vi "Main.vi"(7 "GenNet Protocol":refnum<class "GenNet Protocol.lvclass">, 9 "Port Number":u16, 10 "Caller MsgQ":refnum<class "DQMH-GenNet Message Queue.lvclass">, 11 "Module Admin":refnum<class "Delacor_lib_QMH_Cloneable Module Admin.lvclass">) -> ()   [LabVIEW 2020, in "GenNet-Server.lvlib"]
doc: "The GenNet-Server module is instantiated from a DQMH Generic Networking Module\nin order to accept messages via TCP/IP. \n\nThe GenNet-Server module accepts messages from any DQMH Generic Networking \nModule running in another application and/or on another PC.\n\n<b>Note:</b> This VI was modified by the <b>Validate DQMH Module</b> tool to upgrade it to the DQMH 5.0 approach to destroying cloneable module event references.\n\n<b>Note:</b> This VI was modified by the <b>Validate DQMH Module</b> tool to have the module name be passed as the Additional Information parameter with an Error Reported broadcast.\n\n<b>Note:</b> This VI was modified by the <b>Validate DQMH Module</b> tool to call the Release Message Queue VI in the top-level Error case.\n\n<b>Note:</b> This VI was modified by the <b>Validate DQMH Module</b> tool to call the Release Message Queue VI in the top-level Error case.\n\n<b>Note:</b> This VI was modified by the <b>Validate DQMH Module</b> tool to add a call to the Error Reported VI at the end of the 'Exit' MHL frame.\n\n____\nHAMPEL SOFTWARE ENGINEERING v3.8.0 (2023-12-18 14:41)"
uses:
  GenNet-Server.lvlib
  <vilib>/Delacor/Delacor QMH/Libraries/Cloneable Module Admin_class/Delacor_lib_QMH_Cloneable Module Admin.lvclass
  C:/Program Files (x86)/National Instruments/LabVIEW 2020/vi.lib/Delacor/Delacor QMH/Libraries/Module Admin_class/Delacor_lib_QMH_Module Admin.lvclass
  DQMH-GenNet Message Queue.lvclass
  GenNet Protocols/GenNet Protocol.lvclass
  SubVIs/TCP_Comm-States.ctl
  UDP Broadcasting/Generic Broadcasts.ctl
  hse-dqmh/Dynamic Requesters/Singleton/Status Updated Argument--cluster.ctl
  hse-dqmh/Dynamic Requesters/Singleton/Error Reported Argument--cluster.ctl
  hse-dqmh/Dynamic Requesters/Singleton/Get Module Execution Status Argument--cluster.ctl
  hse-dqmh/Dynamic Requesters/Singleton/Stop Argument--cluster.ctl
  hse-dqmh/Controls/System Message Argument--cluster.ctl
  hse-dqmh/Controls/System Message Source.ctl
  Module Data--cluster.ctl
  UDP Broadcasting/Network Broadcast Params.ctl
  Stop Argument--cluster.ctl
  <vilib>/Delacor/Delacor QMH/Libraries/Message Queue_class/Delacor_lib_QMH_Message Queue.lvclass/Delacor_lib_QMH_Message Queue.ctl
  UDP Broadcasting/Broadcast Arguments/Error Reported - Arguments.ctl
  UDP Broadcasting/Broadcast Arguments/Module Did Stop - Arguments.ctl
  Forward Generic Broadcasts to Network Argument--cluster.ctl
  <vilib>/Delacor/Delacor QMH/Libraries/Cloneable Module Admin_class/Delacor_lib_QMH_Cloneable Module Admin.lvclass/Delacor_lib_QMH_Cloneable Module Admin.ctl
  <vilib>/Delacor/Delacor QMH/Libraries/Module Admin_class/Delacor_lib_QMH_Module Admin.lvclass/Delacor_lib_QMH_Module Admin.ctl
  <vilib>/Utility/miscctls.llb/LVPointTypeDef.ctl
  <vilib>/Delacor/Delacor QMH/Libraries/Cloneable Module Admin_class/Delacor_lib_QMH_Get Module ID.vi
  <vilib>/Delacor/Delacor QMH/Libraries/Message Queue_class/Delacor_lib_QMH_Enqueue Message (Single).vi
  <vilib>/Delacor/Delacor QMH/Libraries/Module Admin_class/Delacor_lib_QMH_Get External Launch.vi
  <vilib>/Utility/tcp.llb/UDP Multicast Write-Only Open.vi
  <vilib>/Utility/error.llb/Error Cluster From Error Code.vi
  <vilib>/ErrorRing/Error Ring.xnode
  <vilib>/Delacor/Delacor QMH/Libraries/Message Queue_class/Delacor_lib_QMH_Message Queue.lvclass
  hse-dqmh/hse-dqmh.lvlib
  hse-gennet.lvlib
  hse-dqmh/hse-dqmh-dynamicrequesters.lvlib
panel:
  out "listener ID":refnum<k5>
  out "error out":errorcluster
  # "The GenNet Protocol allows for injecting the actual protocol (or, rather, the format\nor encoding used for the TCP messages). This also defines how to handle incoming\nmessages (eg. write them directly to the Caller MsgQ or broadcast them)"
  # "The GenNet-Server module is instantiated from a DQMH Generic Networking Module\n(the caller) in order to accept messages via TCP/IP. \n\nThe GenNet-Server module accepts messages from any DQMH Generic Networking \nModule running in another application and/or on another PC."
  # "Caveat:\nThe Caller's message queue, which should be private to the caller only, is avail-\nable to the GenNet-Server module so that it can write messages directly. As the GenNet-Server\nmodule cannot be accessed from other code, and as messages that arrive via\nnetwork are to be considered local, this excemption to the rule is tolerable."
  # "Please get in touch with us at office@hampel-soft.com or visit our website www.hampel-soft.com"
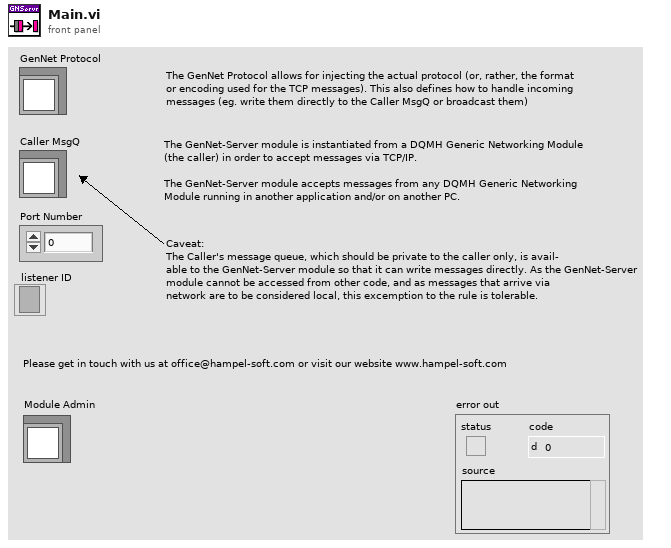
[diagram p1: front panel]
types:
  T1 = typedef "hse-gennet.lvlib/Generic Broadcasts.ctl" = cluster{"Status Updated":refnum<user-event>, "Error Reported":refnum<user-event>, "Update Module Execution Status":refnum<user-event>, "Module Did Stop":refnum<user-event>, "System Message":refnum<user-event>}
  T2 = typedef "GenNet-Server.lvlib/TCP_Comm-States.ctl" = enum16{"Idle", "Open port", "Wait for connection...", "Close port"}
  T3 = typedef "GenNet-Server.lvlib/Request Events--cluster.ctl" = cluster{"Stop Module":refnum<user-event>, "Show Panel":refnum<user-event>, "Hide Panel":refnum<user-event>, "Show Diagram":refnum<user-event>, "Get Module Execution Status":refnum<user-event>, "Forward Generic Broadcasts to Network":refnum<user-event>}
  T4 = typedef "GenNet-Server.lvlib/Module Data--cluster.ctl" = cluster{"Status":string, "UDP Conn. ID":refnum<k16>, "Network Broadcast Params":T5}
  T5 = typedef "hse-gennet.lvlib/Network Broadcast Params.ctl" = cluster{"Server (Sender) Port":u16, "Client (Receiver) Port":u16, "Multicast Address":string, "Local IP Address":string, "Max Rx Byte Size":i32}
  T6 = enum32{"invalid lock state", "Not Locked", "Locked (No Password)", "Password-protected"}
  T7 = typedef "GenNet-Server.lvlib/Stop Argument--cluster.ctl" = cluster{"Origin":string, "Module ID":i32, "Exit via Stop Module Req?":bool, "Wait for Module to stop?":bool}
  T8 = typedef "hse-gennet.lvlib/Error Reported - Arguments.ctl" = cluster{"Error":errorcluster, "Additional Information":string, "Module Name":string}
  T9 = typedef "hse-gennet.lvlib/Module Did Stop - Arguments.ctl" = cluster{"Origin":string, "Exit via Stop Module Req?":bool, "Wait for Module to stop?":bool}
  T10 = typedef "hse-dqmh.lvlib/System Message Source.ctl" = enum16{"module", "application", "network"}
  T11 = typedef "hse-dqmh.lvlib/System Message Argument--cluster.ctl" = cluster{"Identifier":string, "Payload":variant, "Sys. Msg. Source":T10, "Sys. Msg. Origin":string}
  T12 = typedef "GenNet-Server.lvlib/Forward Generic Broadcasts to Network Argument--cluster.ctl" = cluster{"Module ID":i32, "Generic Broadcast Events":T1, "Network Broadcast Params":T5}
  T13 = typedef "LVPointTypeDef.ctl" = cluster{"Horizontal":i16, "Vertical":i16}
  T14 = enum32{"Invalid", "Standard", "Closed", "Hidden", "Minimized", "Maximized"}
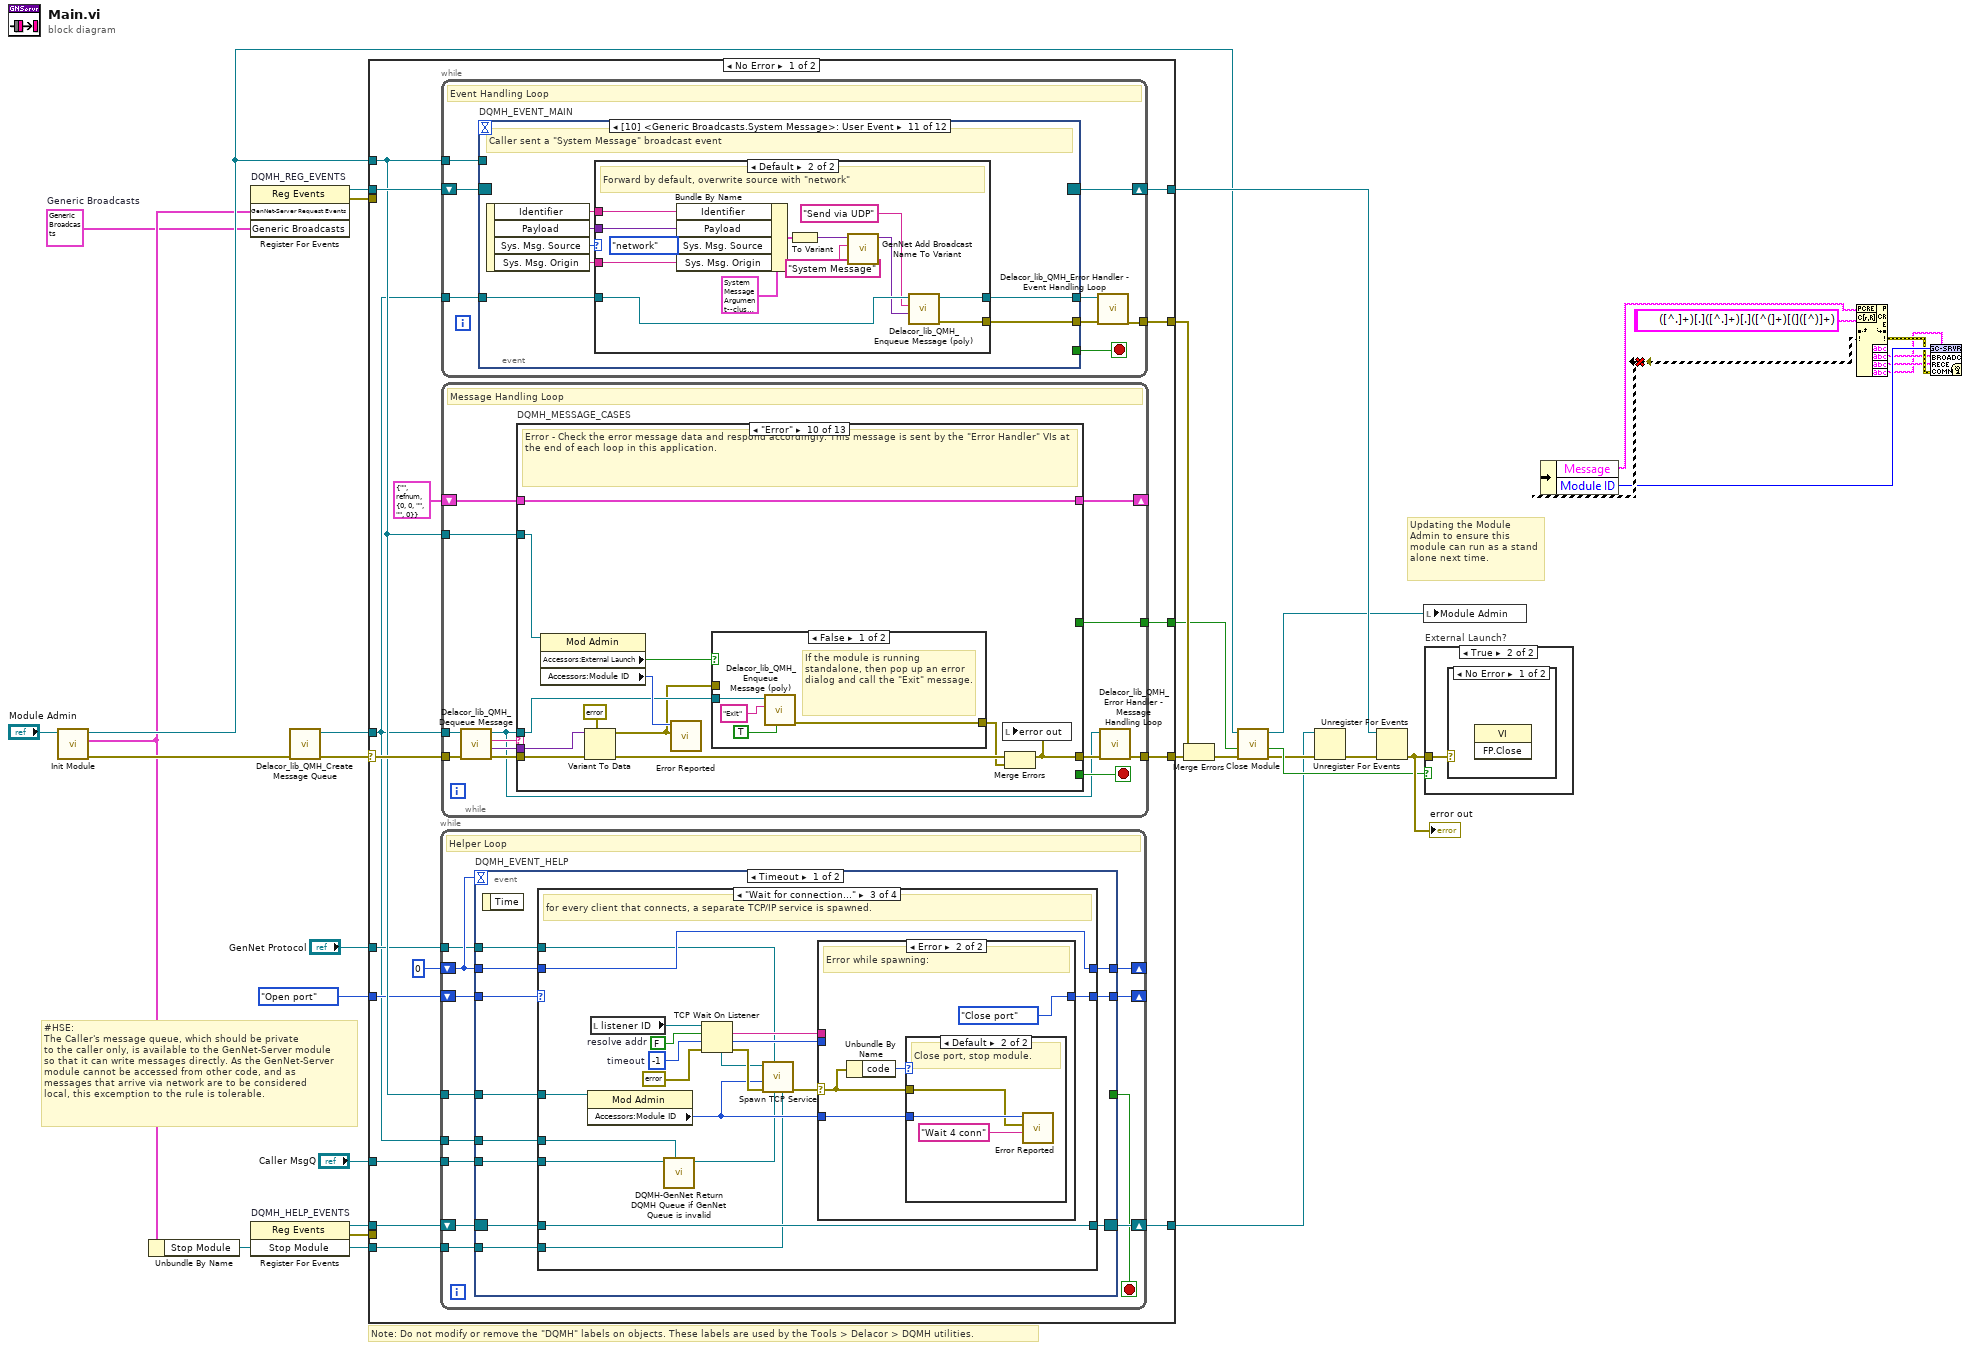
[diagram p0: block diagram]
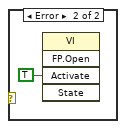
[diagram p3: hidden frame]
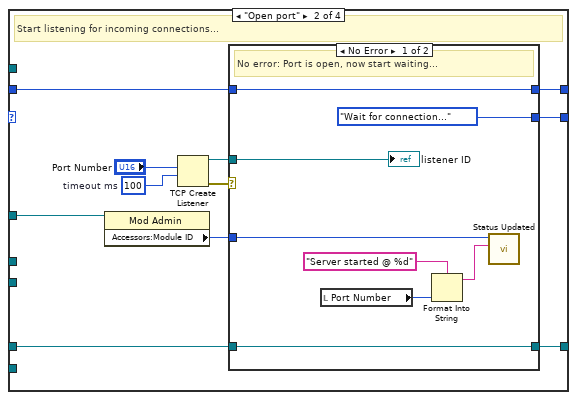
[diagram p5: hidden frame]
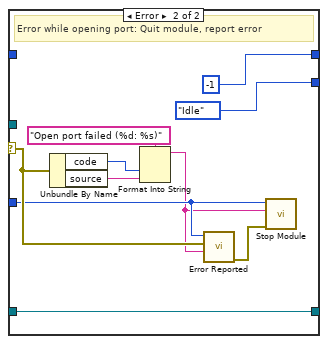
[diagram p6: hidden frame]
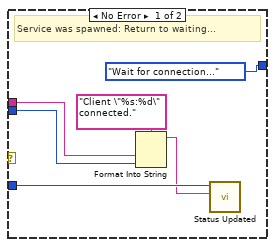
[diagram p7: hidden frame]
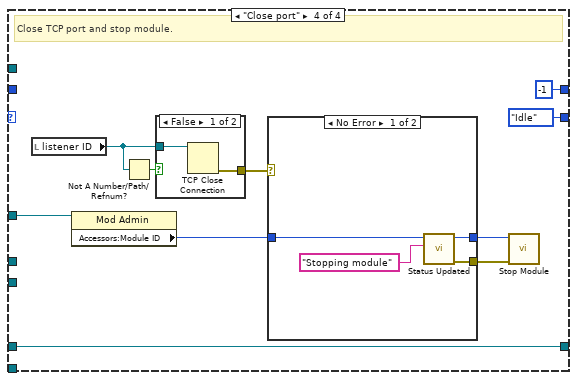
[diagram p9: hidden frame]
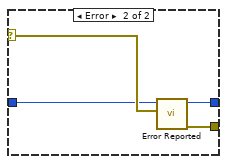
[diagram p11: hidden frame]
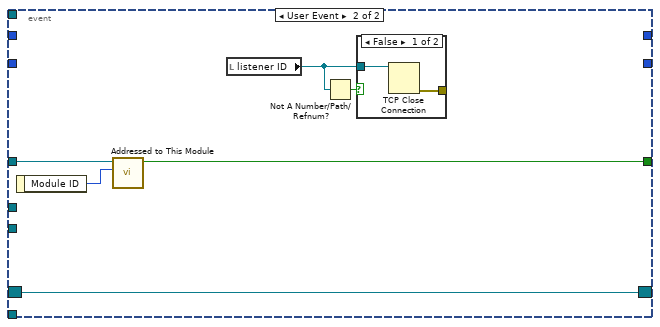
[diagram p12: hidden frame]
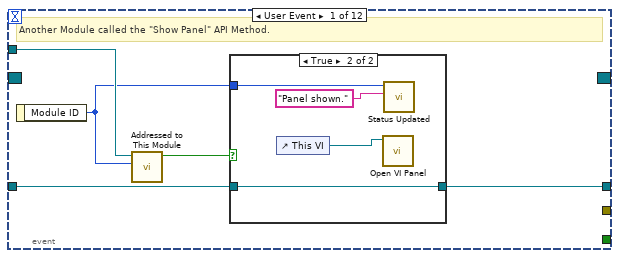
[diagram p14: hidden frame]
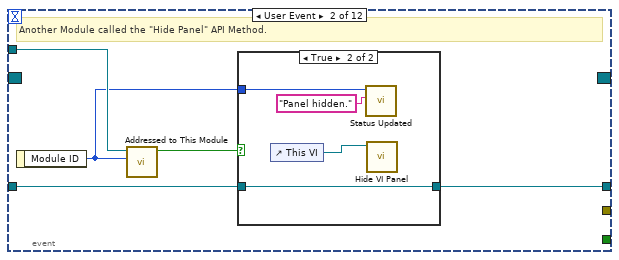
[diagram p16: hidden frame]
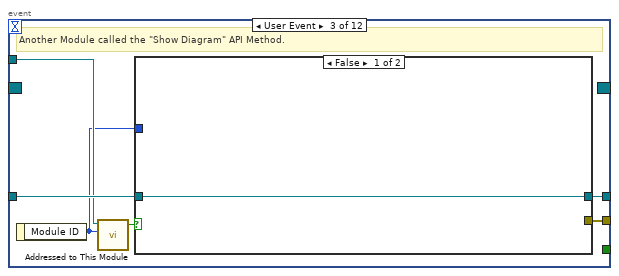
[diagram p18: hidden frame]
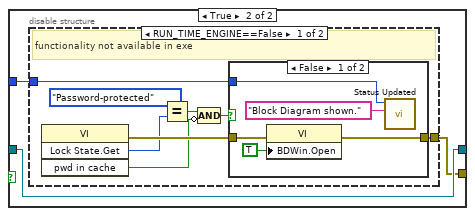
[diagram p19: hidden frame]
diagram:
  w2 = T1 {"Status Updated"=refnum, "Error Reported"=refnum, "Update Module Execution Status"=refnum, "Module Did Stop"=refnum, "System Message"=refnum}  # Generic Broadcasts
  # "#HSE: \nThe Caller's message queue, which should be private \nto the caller only, is available to the GenNet-Server module \nso that it can write messages directly. As the GenNet-Server\nmodule cannot be accessed from other code, and as \nmessages that arrive via network are to be considered \nlocal, this excemption to the rule is tolerable."
  # "Note: Do not modify or remove the \"DQMH\" labels on objects. These labels are used by the Tools > Delacor > DQMH utilities."
  # "Updating the Module Admin to ensure this module can run as a stand alone next time."
  n1 = call "Init Module.vi"("Cloneable Module Admin in"="Module Admin") -> ("error out"=w23:errorcluster, "GenNet-Server Request Events"=w7:T3, "Cloneable Module Admin out"=w18:refnum<class "Delacor_lib_QMH_Cloneable Module Admin.lvclass">)  [unwired: 8 in]
  n2 = Unbundle By Name(w7) -> ("Stop Module"=w6:refnum<user-event>)
  n3 = register-events "DQMH_REG_EVENTS"(w7, w2) -> (reference out=w21:refnum<event-registration>, error out=w4:errorcluster)  [unwired: 2 in]
  n4 = register-events "DQMH_HELP_EVENTS"(w6) -> (reference out=w12:refnum<event-registration>, error out=w3:errorcluster)  [unwired: 2 in]
  n5 = call <vilib>:"Delacor_lib_QMH_Create Message Queue.vi"("error in"=w23) -> ("error out"=w13:errorcluster, "Message Queue"=w20:refnum<class "Delacor_lib_QMH_Message Queue.lvclass">)  [unwired: 9 in]
  n6 = case shown="No Error" w13 {
    selector: w13 -> [w37 w494]
    tunnel: [w42 w494] -> w24
    tunnel: [w41 w495] -> w22
    tunnel: w21 -> [w39 w495]
    tunnel: w20 -> [w27 w486]
    tunnel: [w38 _] -> w25
    tunnel: w18 -> [w34 w490]
    tunnel: [w36 _] -> w16
    tunnel: w12 -> [w35 w487]
    tunnel: "Caller MsgQ" -> [w33 w485]
    tunnel: [w32 w487] -> w8
    tunnel: w6 -> [w30 _]
    tunnel: TCP_Comm-States."Open port" ("comm-states") -> [w29 _]
    tunnel: w4 -> [_ _]
    tunnel: w3 -> [_ _]
    tunnel: "GenNet Protocol" -> [w28 _]
    frame No Error {
      n7 = while {
        shift-right: [w53] -> _
        shift-left: 0 -> [w54]
        tunnel: w34 -> [w52]
        tunnel: w33 -> [w51]
        shift-right: [w48] -> _
        shift-left: w29 -> [w49]
        shift-right: [w50] -> w32
        shift-left: w35 -> [w46]
        tunnel: w30 -> [w45]
        tunnel: w28 -> [w44]
        tunnel: w27 -> [w43]
        stop <- w47 stop-if-true
        # "Helper Loop"
        n8 = event "DQMH_EVENT_HELP" shown="[0] Timeout" {
          selector: w46 -> [w59 w150]
          dyn-events: [w58 w150] -> w50
          timeout: w54 -> [_ _]
          tunnel: w54 -> [w64 _]
          tunnel: [w63 _] -> w53
          tunnel: w52 -> [w62 w153]
          tunnel: w51 -> [w60 _]
          tunnel: w49 -> [w65 _]
          tunnel: [w61 _] -> w48
          tunnel: [_ w151] -> w47
          tunnel: w45 -> [w57 _]
          tunnel: w44 -> [w56 _]
          tunnel: w43 -> [w55 _]
          event Timeout {
            n9 = event-data() -> ()  [unwired: 1 in, 1 out]
            n10 = case shown="\"Wait for connection...\"" w65 {
              selector: w65 -> [w68 _ _ _]
              tunnel: w64 -> [w67 w73 w102 _]
              tunnel: [w67 w72 w102 -1] -> w63
              tunnel: w62 -> [_ w75 w113 w139]
              tunnel: [w68 w79 w109 TCP_Comm-States."Idle" ("comm-states")] -> w61
              tunnel: w60 -> [_ _ w98 _]
              tunnel: w59 -> [w66 w71 w108 w133]
              tunnel: [w66 w70 w108 w133] -> w58
              tunnel: w57 -> [_ _ w107 _]
              tunnel: w56 -> [_ _ w101 _]
              tunnel: w55 -> [_ _ w99 _]
              frame "Idle", Default {
              }
              frame "Open port" {
                w78 = 100  # timeout ms
                # "Start listening for incoming connections..."
                n11 = property class="Mod Admin"(reference=w75) -> ("Accessors:Module ID"=w74:i32)  [unwired: 1 in, 2 out]
                n12 = TCP Create Listener(9:w78, 10:"Port Number") -> (0:w77:errorcluster, 3:w76:refnum<k5>)  [unwired: 3 in, 1 out]
                n13 = case shown="No Error" w77 {
                  selector: w77 -> [_ w91]
                  tunnel: [TCP_Comm-States."Wait for connection..." ("comm-states") TCP_Comm-States."Idle" ("comm-states")] -> w79
                  tunnel: w76 -> [w85 _]
                  tunnel: w74 -> [w81 w90]
                  tunnel: w73 -> [w86 _]
                  tunnel: [w86 -1] -> w72
                  tunnel: w71 -> [w84 w95]
                  tunnel: [w84 w95] -> w70
                  frame No Error {
                    # "No error: Port is open, now start waiting..."
                    n14 = local read "Port Number"() -> (w82:u16)
                    n15 = Format Into String(format string="Server started @ %d" ("Status"), w82) -> (resulting string=w80:string)  [unwired: 2 in, 1 out]
                    n16 = call "Status Updated.vi"("Status"=w80, "Module ID"=w81) -> ()  [unwired: 9 in, 1 out]
                    "listener ID" <- w85
                  }
                  frame Error {
                    # "Error while opening port: Quit module, report error"
                    n17 = Unbundle By Name(w91) -> ("code"=w92:i32, "source"=w93:string)
                    n18 = Format Into String(format string="Open port failed (%d: %s)" ("Origin"), w92, w93) -> (resulting string=w88:string)  [unwired: 2 in, 1 out]
                    n19 = call "Error Reported.vi"("Additional Information"=w88, "Error"=w91, "Module ID"=w90) -> ("error out"=w89:errorcluster)  [unwired: 8 in]
                    n20 = call "Stop Module.vi"("error in (no error)"=w89, "Origin"=w88, "Module ID"=w90) -> ()  [unwired: 8 in, 1 out]
                  }
                }
              }
              frame "Wait for connection..." {
                w104 = FALSE  # resolve addr
                w116 = -1  # timeout
                # "for every client that connects, a separate TCP/IP service is spawned."
                n21 = property class="Mod Admin"(reference=w113) -> ("Accessors:Module ID"=w111:i32)  [unwired: 1 in, 2 out]
                n22 = local read "listener ID"() -> (w110:refnum<k5>)
                n23 = call "DQMH-GenNet Return DQMH Queue if GenNet Queue is invalid.vi"("Message Queue in"=w99, "DQMH-GenNet Message Queue in"=w98) -> ("Message Queue out"=w100:refnum<class "Delacor_lib_QMH_Message Queue.lvclass">)  [unwired: 8 in, 1 out]
                n24 = TCP Wait On Listener(8:errorcluster {"status"=FALSE, "code"=0, "source"=""} ("error in (no error)"), 9:w116, 10:w104, 11:w110) -> (0:w115:errorcluster, 1:w105:u16, 2:w106:string, 4:w114:refnum<k5>)  [unwired: 1 out]
                n25 = call "Spawn TCP Service.vi"("Stop Module"=w107, "Message Queue"=w100, "GenNet Protocol"=w101, "error in"=w115, "Module ID"=w111, "Connection ID"=w114) -> ("error out"=w112:errorcluster)  [unwired: 5 in]
                n26 = case shown="Error" w112 {
                  selector: w112 -> [_ w124]
                  tunnel: w111 -> [w118 w126]
                  tunnel: [TCP_Comm-States."Wait for connection..." ("comm-states") TCP_Comm-States."Close port" ("comm-states")] -> w109
                  tunnel: w106 -> [w120 _]
                  tunnel: w105 -> [w119 _]
                  frame No Error {
                    # "Service was spawned: Return to waiting..."
                    n27 = Format Into String(format string="Client \"%s:%d\" connected.", w120, w119) -> (resulting string=w117:string)  [unwired: 2 in, 1 out]
                    n28 = call "Status Updated.vi"("Status"=w117, "Module ID"=w118) -> ()  [unwired: 9 in, 1 out]
                  }
                  frame Error {
                    # "Error while spawning:"
                    n29 = Unbundle By Name(w124) -> ("code"=w123:i32)
                    n30 = case shown="Default" w123 {
                      tunnel: w124 -> [_ w128]
                      tunnel: w126 -> [_ w129]
                      frame 66 {
                        # "closed by peer: No error."
                      }
                      frame Default {
                        # "Close port, stop module."
                        n31 = call "Error Reported.vi"("Additional Information"="Wait 4 conn", "Error"=w128, "Module ID"=w129) -> ()  [unwired: 8 in, 1 out]
                      }
                    }
                  }
                }
              }
              frame "Close port" {
                # "Close TCP port and stop module."
                n32 = local read "listener ID"() -> (w134:refnum<k5>)
                n33 = property class="Mod Admin"(reference=w139) -> ("Accessors:Module ID"=w132:i32)  [unwired: 1 in, 2 out]
                n34 = Not A Number/Path/Refnum?(number/path/refnum=w134) -> (NaN/Path/Refnum?=w136:bool)
                n35 = case shown="False" w136 {
                  tunnel: [w141 _] -> w135
                  tunnel: w134 -> [w140 _]
                  frame False {
                    n36 = TCP Close Connection(connection ID=w140) -> (error out=w141:errorcluster)  [unwired: 2 in, 1 out]
                  }
                  frame True {
                  }
                }
                n37 = case shown="No Error" w135 {
                  selector: w135 -> [_ w147]
                  tunnel: w132 -> [w143 w145]
                  tunnel: [w144 w146] -> w131
                  tunnel: [w143 w145] -> w130
                  frame No Error {
                    n38 = call "Status Updated.vi"("Status"="Stopping module", "Module ID"=w143) -> ("error out"=w144:errorcluster)  [unwired: 9 in]
                  }
                  frame Error {
                    n39 = call "Error Reported.vi"("Error"=w147, "Module ID"=w145) -> ("error out"=w146:errorcluster)  [unwired: 9 in]
                  }
                }
                n40 = call "Stop Module.vi"("error in (no error)"=w131, "Module ID"=w130) -> ()  [unwired: 9 in, 1 out]
              }
            }
          }
          event User Event {
            n41 = event-data() -> ("Module ID"=w152:i32)  [unwired: 1 in]
            n42 = call "Addressed to This Module.vi"("Module ID from Argument"=w152, "Module Admin"=w153) -> ("Addressed to this instance?"=w151:bool)  [unwired: 8 in, 1 out]
            n43 = local read "listener ID"() -> (w148:refnum<k5>)
            n44 = Not A Number/Path/Refnum?(number/path/refnum=w148) -> (NaN/Path/Refnum?=w149:bool)
            n45 = case shown="False" w149 {
              tunnel: [w155 _] -> _
              tunnel: w148 -> [w154 _]
              frame False {
                n46 = TCP Close Connection(connection ID=w154) -> (error out=w155:errorcluster)  [unwired: 2 in, 1 out]
              }
              frame True {
              }
            }
          }
        }
      }
      n47 = while {
        tunnel: w27 -> [w163]
        shift-right: [w161] -> w41
        shift-left: w39 -> [w162]
        tunnel: [w157] -> w38
        tunnel: w34 -> [w156]
        stop <- w159 stop-if-true
        # "Event Handling Loop"
        n48 = event "DQMH_EVENT_MAIN" shown="[10] <Generic Broadcasts.System Message>: User Event" {
          selector: w162 -> [_ _ _ _ _ _ _ _ _ _ _ w308]
          dyn-events: [_ _ _ _ _ _ _ _ _ _ _ w309] -> w161
          timeout: _ -> [_ _ _ _ _ _ _ _ _ _ _ _]
          tunnel: [_ _ _ w212 _ _ _ _ _ _ _ _] -> w159
          tunnel: w163 -> [w168 w178 w189 w215 w235 w239 w251 w264 w270 w283 w291 w315]
          tunnel: [_ _ w184 w217 w234 w238 w249 w261 w269 w281 w289 w311] -> w160
          tunnel: [w167 w177 w188 w216 w233 w239 w250 w262 w271 w282 w290 w314] -> w158
          tunnel: w156 -> [w165 w175 w186 w214 _ w240 _ _ _ _ _ w312]
          event User Event {
            # "Another Module called the \"Show Panel\" API Method."
            n49 = event-data() -> ("Module ID"=w164:i32)  [unwired: 1 in]
            n50 = call "Addressed to This Module.vi"("Module ID from Argument"=w164, "Module Admin"=w165) -> ("Addressed to this instance?"=w166:bool)  [unwired: 8 in, 1 out]
            n51 = case shown="True" w166 {
              tunnel: w168 -> [w169 w173]
              tunnel: [w169 w173] -> w167
              tunnel: w164 -> [_ w171]
              frame False {
              }
              frame True {
                n52 = control-ref of="This VI"() -> (w170:refnum<vi>)
                n53 = call "Open VI Panel.vi"("VI"=w170) -> ()  [unwired: 10 in, 1 out]
                n54 = call "Status Updated.vi"("Status"="Panel shown." ("format string"), "Module ID"=w171) -> ()  [unwired: 9 in, 1 out]
              }
            }
          }
          event User Event {
            # "Another Module called the \"Hide Panel\" API Method."
            n55 = event-data() -> ("Module ID"=w174:i32)  [unwired: 1 in]
            n56 = call "Addressed to This Module.vi"("Module ID from Argument"=w174, "Module Admin"=w175) -> ("Addressed to this instance?"=w176:bool)  [unwired: 8 in, 1 out]
            n57 = case shown="True" w176 {
              tunnel: w178 -> [w179 w183]
              tunnel: [w179 w183] -> w177
              tunnel: w174 -> [_ w181]
              frame False {
              }
              frame True {
                n58 = control-ref of="This VI"() -> (w180:refnum<vi>)
                n59 = call "Status Updated.vi"("Status"="Panel hidden." ("format string"), "Module ID"=w181) -> ()  [unwired: 9 in, 1 out]
                n60 = call "Hide VI Panel.vi"("VI"=w180) -> ()  [unwired: 10 in, 1 out]
              }
            }
          }
          event User Event {
            # "Another Module called the \"Show Diagram\" API Method."
            n61 = event-data() -> ("Module ID"=w185:i32)  [unwired: 1 in]
            n62 = call "Addressed to This Module.vi"("Module ID from Argument"=w185, "Module Admin"=w186) -> ("Addressed to this instance?"=w187:bool)  [unwired: 8 in, 1 out]
            n63 = case shown="False" w187 {
              tunnel: w189 -> [w190 w192]
              tunnel: [w190 w192] -> w188
              tunnel: w185 -> [_ w193]
              tunnel: [_ w191] -> w184
              frame False {
              }
              frame True {
                n64 = disable-structure shown="RUN_TIME_ENGINE==False" {
                  disable-tunnel: [w201 errorcluster {"status"=FALSE, "code"=0, "source"=""} ("error out")] -> w191
                  disable-tunnel: w193 -> [w194 _]
                  frame condition #0 (active) {
                    # "functionality not available in exe"
                    n65 = invoke class="VI" method="Lock State.Get"() -> (error out=w200:errorcluster, "Get Lock State"=w199:T6, "pwd in cache"=w196:bool)  [unwired: 4 in, 1 out]
                    n66 = Equal?(x=T6."Password-protected", y=w199) -> (x = y?=w197:bool)
                    n67 = Compound Arithmetic op=AND(w197, invert w196) -> (w195:bool)
                    n68 = case shown="False" w195 {
                      tunnel: [w205 w207] -> w201
                      tunnel: w200 -> [w204 w207]
                      tunnel: w194 -> [w202 _]
                      frame False {
                        n69 = property class="VI"(error in=w204, "BDWin.Open"=TRUE ("Block Diagram Window:Open")) -> (error out=w205:errorcluster)  [unwired: 1 in, 1 out]
                        n70 = call "Status Updated.vi"("Status"="Block Diagram shown." ("format string"), "Module ID"=w202) -> ()  [unwired: 9 in, 1 out]
                      }
                      frame True {
                        # "Password-protected VI, and the password is not in the cache. Do not show the diagram."
                      }
                    }
                  }
                  frame condition #1 {
                  }
                }
              }
            }
          }
          event User Event {
            # "Another Module called the \"Stop Module\" API Method  or the Message Handling Loop below."
            n71 = event-data() -> ("Module ID"=w210:i32, "Wait for Module to stop?"=w211:bool, "Origin"=w209:string)  [unwired: 1 in]
            n72 = call "Addressed to This Module.vi"("Module ID from Argument"=w210, "Module Admin"=w214) -> ("Addressed to this instance?"=w213:bool)  [unwired: 8 in, 1 out]
            n73 = case shown="True" w213 {
              tunnel: [_ w227] -> w217
              tunnel: [w218 w226] -> w216
              tunnel: w215 -> [w218 w225]
              tunnel: [_ TRUE] -> w212
              tunnel: w211 -> [_ w220]
              tunnel: w210 -> [_ w222]
              tunnel: w209 -> [_ _]
              frame False {
              }
              frame True {
                # "The event can get fired from the Exit message. The queue gets destroyed there. In this case, the Enqueue VI will return error 1. It is safe to ignore, because the module is already exiting."
                n74 = Bundle By Name(cluster=T7 {"Origin"="", "Module ID"=-1, "Exit via Stop Module Req?"=FALSE, "Wait for Module to stop?"=FALSE} ("Stop Argument"), "Module ID"=w222, "Exit via Stop Module Req?"=TRUE, "Wait for Module to stop?"=w220) -> (w219:T7)
                n75 = call-poly <vilib>:"Delacor_lib_QMH_Enqueue Message (poly).vi"("Priority Message? (F)"=TRUE, "Message Data"=w219, "Message"="Exit", "Message Queue in"=w225) -> ("error out"=w230:errorcluster, "Message Queue out"=w226:refnum<class "Delacor_lib_QMH_Message Queue.lvclass">)  [unwired: 6 in]
                n76 = call <vilib>:"Clear Errors.vi"("error in (no error)"=w230, "specific error code to clear (0: all)"=1) -> ("error out"=w227:errorcluster)  [unwired: 4 in, 1 out]
              }
            }
          }
          event Panel Close? {
            w236 = TRUE  # Discard the event so the 'Confirm Quit' message has a chance to run.
            # "Send the 'Confirm Quit' message if the user closes the panel of the VI."
            n77 = event-data() -> ()  [unwired: 1 in, 1 out]
            n78 = call-poly <vilib>:"Delacor_lib_QMH_Enqueue Message (poly).vi"("Message"="Confirm Quit", "Message Queue in"=w235) -> ("error out"=w234:errorcluster, "Message Queue out"=w233:refnum<class "Delacor_lib_QMH_Message Queue.lvclass">)  [unwired: 8 in]
            n79 = event-data("Discard?"=w236) -> ()  [unwired: 1 in, 1 out]
          }
          event User Event {
            # "For cloneable running as singleton, broadcast that the module is running."
            n80 = event-data() -> ("Module ID"=w237:i32)  [unwired: 1 in]
            n81 = call "Addressed to This Module.vi"("Module ID from Argument"=w237, "Module Admin"=w240) -> ("Addressed to this instance?"=w241:bool)  [unwired: 8 in, 1 out]
            n82 = case shown="True" w241 {
              tunnel: [_ w244] -> w238
              tunnel: w237 -> [_ w243]
              frame False {
              }
              frame True {
                n83 = call "Update Module Execution Status.vi"("Running?"=TRUE, "Module ID"=w243) -> ("error out"=w244:errorcluster)  [unwired: 9 in]
              }
            }
          }
          event User Event {
            # "Caller sent a \"Status Updated\" broadcast event"
            n84 = event-data() -> ("Status"=w246:string)  [unwired: 1 in]
            n85 = To Variant(anything=w246) -> (Variant=w248:variant)
            n86 = call "GenNet Add Broadcast Name To Variant.vi"("Broadcast Name"="Status Updated", "Broadcast Data IN"=w248) -> ("Variant OUT"=w245:variant)  [unwired: 9 in]
            n87 = call-poly <vilib>:"Delacor_lib_QMH_Enqueue Message (poly).vi"("Message Data"=w245, "Message"="Send via UDP", "Message Queue in"=w251) -> ("error out"=w249:errorcluster, "Message Queue out"=w250:refnum<class "Delacor_lib_QMH_Message Queue.lvclass">)  [unwired: 7 in]
          }
          event User Event {
            # "Caller sent a \"Error reported\" broadcast event"
            n88 = event-data() -> ("Error"=w259:errorcluster, "Additional Information"=w258:string, "Module Name"=w257:string)  [unwired: 1 in]
            n89 = Bundle By Name(cluster=T8 {"Error"={"status"=FALSE, "code"=0, "source"=""}, "Additional Information"="", "Module Name"=""}, "Error"=w259, "Additional Information"=w258, "Module Name"=w257) -> (w254:T8)
            n90 = To Variant(anything=w254) -> (Variant=w256:variant)
            n91 = call "GenNet Add Broadcast Name To Variant.vi"("Broadcast Name"="Error Reported", "Broadcast Data IN"=w256) -> ("Variant OUT"=w253:variant)  [unwired: 9 in]
            n92 = call-poly <vilib>:"Delacor_lib_QMH_Enqueue Message (poly).vi"("Message Data"=w253, "Message"="Send via UDP", "Message Queue in"=w264) -> ("error out"=w261:errorcluster, "Message Queue out"=w262:refnum<class "Delacor_lib_QMH_Message Queue.lvclass">)  [unwired: 7 in]
          }
          event User Event {
            # "Caller sent a \"Update Module Execution Status\" broadcast event"
            n93 = event-data() -> ("Running?"=w266:bool)  [unwired: 1 in]
            n94 = To Variant(anything=w266) -> (Variant=w268:variant)
            n95 = call "GenNet Add Broadcast Name To Variant.vi"("Broadcast Name"="Update Module Execution Status", "Broadcast Data IN"=w268) -> ("Variant OUT"=w265:variant)  [unwired: 9 in]
            n96 = call-poly <vilib>:"Delacor_lib_QMH_Enqueue Message (poly).vi"("Message Data"=w265, "Message"="Send via UDP", "Message Queue in"=w270) -> ("error out"=w269:errorcluster, "Message Queue out"=w271:refnum<class "Delacor_lib_QMH_Message Queue.lvclass">)  [unwired: 7 in]
          }
          event User Event {
            # "Caller sent a \"Module Did Stop\" broadcast event"
            n97 = event-data() -> ("Origin"=w280:string, "Exit via Stop Module Req?"=w278:bool, "Wait for Module to stop?"=w279:bool)  [unwired: 1 in]
            n98 = Bundle By Name(cluster=T9 {"Origin"="", "Exit via Stop Module Req?"=FALSE, "Wait for Module to stop?"=FALSE} ("Module Did Stop - Arguments"), "Origin"=w280, "Exit via Stop Module Req?"=w278, "Wait for Module to stop?"=w279) -> (w274:T9)
            n99 = To Variant(anything=w274) -> (Variant=w277:variant)
            n100 = call "GenNet Add Broadcast Name To Variant.vi"("Broadcast Name"="Module Did Stop", "Broadcast Data IN"=w277) -> ("Variant OUT"=w273:variant)  [unwired: 9 in]
            n101 = call-poly <vilib>:"Delacor_lib_QMH_Enqueue Message (poly).vi"("Message Data"=w273, "Message"="Send via UDP", "Message Queue in"=w283) -> ("error out"=w281:errorcluster, "Message Queue out"=w282:refnum<class "Delacor_lib_QMH_Message Queue.lvclass">)  [unwired: 7 in]
          }
          event User Event {
            # "Caller sent a \"System Message\" broadcast event"
            n102 = event-data() -> ("Identifier"=w288:string, "Payload"=w287:variant, "Sys. Msg. Source"=w286:T10, "Sys. Msg. Origin"=w285:string)  [unwired: 1 in]
            n103 = case shown="Default" w286 {
              tunnel: w291 -> [w292 w305]
              tunnel: [w292 w303] -> w290
              tunnel: [_ w302] -> w289
              tunnel: w288 -> [_ w301]
              tunnel: w287 -> [_ w300]
              tunnel: w285 -> [_ w294]
              frame "network" {
                # "Do not forward if originally received via network"
              }
              frame Default {
                # "Forward by default, overwrite source with \"network\""
                n104 = Bundle By Name(cluster=T11 {"Identifier"="", "Payload"=variant, "Sys. Msg. Source"=enum."module", "Sys. Msg. Origin"=""} ("System Message Argument"), "Identifier"=w301, "Payload"=w300, "Sys. Msg. Source"=System_Message_Source."network" ("Source"), "Sys. Msg. Origin"=w294) -> (w299:T11)
                n105 = To Variant(anything=w299) -> (Variant=w298:variant)
                n106 = call "GenNet Add Broadcast Name To Variant.vi"("Broadcast Name"="System Message", "Broadcast Data IN"=w298) -> ("Variant OUT"=w297:variant)  [unwired: 9 in]
                n107 = call-poly <vilib>:"Delacor_lib_QMH_Enqueue Message (poly).vi"("Message Data"=w297, "Message"="Send via UDP", "Message Queue in"=w305) -> ("error out"=w302:errorcluster, "Message Queue out"=w303:refnum<class "Delacor_lib_QMH_Message Queue.lvclass">)  [unwired: 7 in]
              }
            }
          }
          event User Event {
            # "Another Module called the \"Forward Generic Broadcasts to Network\" API Method."
            n108 = event-data() -> ("Generic Broadcast Events"=w307:T1, "Network Broadcast Params"=w306:T5, "Module ID"=w310:i32)  [unwired: 1 in]
            n109 = call "Addressed to This Module.vi"("Module ID from Argument"=w310, "Module Admin"=w312) -> ("Addressed to this instance?"=w313:bool)  [unwired: 8 in, 1 out]
            n110 = case shown="True" w313 {
              tunnel: w315 -> [w317 w327]
              tunnel: [w317 w326] -> w314
              tunnel: [_ w324] -> w311
              tunnel: [w316 w323] -> w309
              tunnel: w308 -> [w316 w322]
              tunnel: w307 -> [_ w321]
              tunnel: w306 -> [_ w320]
              frame False {
              }
              frame True {
                n111 = Bundle By Name(cluster=T12 {"Module ID"=-1, "Generic Broadcast Events"={"Status Updated"=refnum, "Error Reported"=refnum, "Update Module Execution Status"=refnum, "Module Did Stop"=refnum, "System Message"=refnum}, "Network Broadcast Params"={"Server (Sender) Port"=0, "Client (Receiver) Port"=0, "Multicast Address"="", "Local IP Address"="", "Max Rx Byte Size"=0}} ("Forward Generic Broadcasts to Network Argument"), "Network Broadcast Params"=w320) -> (w319:T12)
                n112 = register-events "DQMH_REG_INNER"(reference=w322, w321) -> (reference out=w323:refnum<event-registration>)  [unwired: 2 in, 1 out]
                n113 = call-poly <vilib>:"Delacor_lib_QMH_Enqueue Message (poly).vi"("Message Data"=w319, "Message"="Create UDP Sender", "Message Queue in"=w327) -> ("error out"=w324:errorcluster, "Message Queue out"=w326:refnum<class "Delacor_lib_QMH_Message Queue.lvclass">)  [unwired: 7 in]
              }
            }
          }
        }
        n114 = call-dynamic "Delacor_lib_QMH_Error Handler - Event Handling Loop.vi"("error in"=w160, "Message Queue in"=w158) -> ("dup error in"=w157:errorcluster)  [unwired: 8 in, 1 out]
      }
      n115 = while {
        tunnel: w27 -> [w332]
        shift-right: [w338] -> _
        shift-left: T4 {"Status"="", "UDP Conn. ID"=refnum, "Network Broadcast Params"={"Server (Sender) Port"=0, "Client (Receiver) Port"=0, "Multicast Address"="", "Local IP Address"="", "Max Rx Byte Size"=0}} ("Data Cluster") -> [w339]
        tunnel: w37 -> [w336]
        tunnel: [w330] -> w42
        tunnel: w34 -> [w329]
        tunnel: [w328] -> w36
        stop <- w337 stop-if-true
        # "Message Handling Loop"
        n116 = call-dynamic "Delacor_lib_QMH_Dequeue Message.vi"("error in"=w336, "Message Queue in"=w332) -> ("error out"=w335:errorcluster, "Message Data"=w333:variant, "Message"=w334:string, "Message Queue out"=w331:refnum<class "Delacor_lib_QMH_Message Queue.lvclass">)  [unwired: 6 in]
        n117 = case "DQMH_MESSAGE_CASES" shown="\"Error\"" w334 {
          selector: w334 -> [_ _ _ _ _ _ _ _ _ _ _ _ w474]
          tunnel: w331 -> [_ _ _ _ _ _ _ _ _ w421 w438 w464 _]
          tunnel: w335 -> [w350 w363 w370 w385 w401 w406 w410 w415 w418 w430 w437 w466 _]
          tunnel: [w341 w361 w378 w387 w399 w407 w411 w413 w416 w420 w436 w443 w475] -> w340
          tunnel: w339 -> [w349 w362 w376 w386 w400 w408 w412 w414 w417 w429 w441 w445 w476]
          tunnel: [w349 w362 w375 w386 w400 w408 w412 w414 w417 w429 w441 w445 w476] -> w338
          tunnel: [_ _ _ _ _ _ _ _ _ _ _ w463 _] -> w337
          tunnel: w333 -> [_ _ w368 w384 _ w404 _ _ _ w428 _ w458 _]
          tunnel: w329 -> [w345 _ _ _ _ w403 _ _ _ w425 _ w448 w472]
          tunnel: [_ _ _ _ _ _ _ _ _ _ _ w456 _] -> w328
          frame "Initialize" {
            # "\"Create UDP Sender\""
            # "Initialize - Any operation that needs to be done before the module can receive messages. Synchronize Caller Events.vi will inform Start Module.vi that the module has launched and is ready to receive messages. Module Did Init.vi will broadcast that the module initialized."
            n118 = call "Synchronize Caller Events.vi"("error in (no error)"=w350, "Module Admin"=w345) -> ("error out"=w347:errorcluster, "Module Admin out"=w344:refnum<class "Delacor_lib_QMH_Cloneable Module Admin.lvclass">)  [unwired: 8 in]
            n119 = property class="Mod Admin"(reference=w344) -> ("Accessors:Module ID"=w343:i32, "Accessors:External Launch"=w346:bool)  [unwired: 1 in, 2 out]
            n120 = call "Module Name--constant.vi"("Module ID"=w343) -> ("Module Name"=w342:string)  [unwired: 10 in]
            n121 = disable-structure shown="TARGET_TYPE==Windows||EMBEDDED_UI==True" {
              disable-tunnel: w346 -> [w353 _]
              disable-tunnel: w342 -> [w351 _]
              frame condition #0 (active) {
                n122 = property class="VI"("Front Panel.Title"=w351) -> (reference out=w359:refnum<vi>, error out=w360:errorcluster)  [unwired: 2 in]
                n123 = Select(t=T14."Hidden" ("State"), s=w353, f=T14."Standard" ("State")) -> (s? t:f=w354:T14)
                n124 = invoke class="VI" method="FP.Open"(reference=w359, error in=w360, "State"=w354) -> (reference out=w358:refnum<vi>, error out=w357:errorcluster)  [unwired: 2 in, 3 out]
                n125 = invoke class="VI" method="FP.Center"(reference=w358, error in=w357) -> ()  [unwired: 1 in, 3 out]
                n126 = property on="Pane" class="Pane"("Origin"=T13 {"Horizontal"=0, "Vertical"=0}) -> ()  [unwired: 2 in, 2 out]
              }
              frame condition #1 {
              }
            }
            n127 = call "Module Did Init.vi"("error in (no error)"=w347, "Initialized?"=TRUE, "Origin"=w342, "Module ID"=w343) -> ("error out"=w341:errorcluster)  [unwired: 7 in]
          }
          frame "--- UDP Broadcasting ---" {
            # "Separator -- The following cases handle UDP broadcasting."
            n128 = Merge Errors(w363) -> (w361:errorcluster)
          }
          frame "Create UDP Sender" {
            # "Opens a UDP multicast socket for broadcast forwarding"
            n129 = Variant To Data(error in=w370, type=T12 {"Module ID"=-1, "Generic Broadcast Events"={"Status Updated"=refnum, "Error Reported"=refnum, "Update Module Execution Status"=refnum, "Module Did Stop"=refnum, "System Message"=refnum}, "Network Broadcast Params"={"Server (Sender) Port"=0, "Client (Receiver) Port"=0, "Multicast Address"="", "Local IP Address"="", "Max Rx Byte Size"=0}} ("Forward Generic Broadcasts to Network Argument"), Variant=w368) -> (data=w367:T12, error out=w369:errorcluster)
            n130 = Unbundle By Name(w367) -> ("Network Broadcast Params.Local IP Address"=w364:string, "Network Broadcast Params.Server (Sender) Port"=w371:u16)
            n131 = Unbundle By Name(w367) -> ("Network Broadcast Params"=w366:T5)
            n132 = String To IP(1:w364) -> (0:w377:u32)
            n133 = call-poly <vilib>:"UDP Multicast Open.vi"("net address"=w377, "error in (no error)"=w369, "port"=w371) -> ("error out"=w373:errorcluster, "connection ID"=w374:refnum<k16>)  [unwired: 7 in]
            n134 = Bundle By Name(cluster=w376, "Network Broadcast Params"=w366, "UDP Conn. ID"=w374) -> (w375:T4)
            n135 = Format Into String(format string="Create UDP Sender on Port %d" ("Message"), w371) -> ()  [unwired: 2 in, 2 out]
            n136 = Merge Errors(w373) -> (w378:errorcluster)
          }
          frame "Send via UDP" {
            # "Forwards the broadcast events of the caller via UDP"
            n137 = Unbundle By Name(w386) -> ("Network Broadcast Params.Multicast Address"=w380:string, "Network Broadcast Params.Client (Receiver) Port"=w379:u16, "UDP Conn. ID"=w382:refnum<k16>)
            n138 = Not A Number/Path/Refnum?(number/path/refnum=w382) -> (NaN/Path/Refnum?=w381:bool)
            n139 = case shown="False" w381 {
              tunnel: w385 -> [w397 w398]
              tunnel: [w388 w398] -> w383
              tunnel: w382 -> [w395 _]
              tunnel: w380 -> [w391 _]
              tunnel: w379 -> [w390 _]
              tunnel: w384 -> [w394 _]
              frame False {
                # "Send via UDP"
                n140 = call "GenNet Send UDP Message.vi"("Multicast IP Address"=w391, "timeout [ms]"=1000, "Receiver Port"=w390, "error in (no error)"=w397, "Message Data"=w394, "UDP Network Connection in"=w395) -> ("error out"=w389:errorcluster)  [unwired: 4 in, 1 out]
                n141 = call "GenNet Get Broadcast Name From Variant.vi"("error in"=w389, "Broadcast Data IN"=w394) -> ("error out"=w388:errorcluster, "Broadcast Name"=w392:string)  [unwired: 7 in, 1 out]
                n142 = Format Into String(format string="Send Broadcast \"%s\" via UDP to IP %s and Port %d" ("Message"), w392, w391, w390) -> ()  [unwired: 2 in, 2 out]
              }
              frame True {
                (unwired) "Send via UDP: Invalid UDP Connection ID" ("Message")
                # "Invalid ID"
              }
            }
            n143 = Merge Errors(w383) -> (w387:errorcluster)
          }
          frame "--- GenNet ---" {
            # "Separator -- The following cases handle messages specific to this Module."
            n144 = Merge Errors(w401) -> (w399:errorcluster)
          }
          frame "GenNet Message Received" {
            # "Forwards a received GenNet message via the corresponding broadcast. The GenNet Protocol \"Process Message\" method decides whether this MHL case is used to broadcast GenNet messages."
            n145 = property class="Mod Admin"(reference=w403) -> ("Accessors:Module ID"=w402:i32)  [unwired: 1 in, 2 out]
            n146 = call "GenNet Message Received.vi"("error in"=w406, "Message"=w404, "Module ID"=w402) -> ("error out"=w405:errorcluster)  [unwired: 8 in]
            n147 = Merge Errors(w405) -> (w407:errorcluster)
          }
          frame "System Message" {
            w409 = "sys msg!"  # message
            # "ignore \"system message\" broadcast for the time being..."
            # "When not wiring the Caller MsgQ, GenNet-Server will instead use its own, local message queue.\n--> receives the \"System Message\" broadcast message"
            n148 = One Button Dialog(message=w409) -> ()  [unwired: 1 in, 1 out]
            n149 = Merge Errors(w410) -> (w411:errorcluster)
          }
          frame "---Copy This Frame---" {
            # "Duplicate this frame when creating new messages.  Change this comment in the duplicated frame to describe this message."
            n150 = Merge Errors(w415) -> (w413:errorcluster)
          }
          frame "--- Exit and Error Handling---" {
            # "Separator - the following cases handle errors and exit messages."
            n151 = Merge Errors(w418) -> (w416:errorcluster)
          }
          frame "Error" {
            # "Error - Check the error message data and respond accordingly. This message is sent by the \"Error Handler\" VIs at the end of each loop in this application."
            n152 = property class="Mod Admin"(reference=w425) -> ("Accessors:External Launch"=w422:bool, "Accessors:Module ID"=w424:i32)  [unwired: 1 in, 2 out]
            n153 = Variant To Data(error in=w430, type=errorcluster {"status"=FALSE, "code"=0, "source"=""} ("error constant"), Variant=w428) -> (data=w419:errorcluster, error out=w426:errorcluster)
            n154 = call "Error Reported.vi"("Error"=w419, "Module ID"=w424) -> ()  [unwired: 9 in, 1 out]
            n155 = case shown="False" w422 {
              tunnel: [w434 _] -> w423
              tunnel: w421 -> [w433 _]
              tunnel: w419 -> [_ _]
              frame False {
                # "If the module is running standalone, then pop up an error dialog and call the \"Exit\" message."
                n156 = call-poly <vilib>:"Delacor_lib_QMH_Enqueue Message (poly).vi"("Priority Message? (F)"=TRUE, "Message"="Exit", "Message Queue in"=w433) -> ("error out"=w434:errorcluster)  [unwired: 7 in, 1 out]
              }
              frame True {
                # "If the module was launched externally, calling the Error Reported broadcast VI is the only action performed by the \"Error\" message. The module's caller can then process the error appropriately."
              }
            }
            n157 = Merge Errors(w426, w423) -> (w420:errorcluster)
            n158 = local write "error out"(w420) -> ()
          }
          frame "Confirm Quit" {
            # "#CodeNeeded - If you want to provide an \"Are you sure\" dialog (or some other notification) before the application exits, place that code here. This message is typically sent from a Panel Close? event."
            # "Confirm Quit - Message that can confirm whether or not the user wants to exit this instance."
            n159 = call-poly <vilib>:"Delacor_lib_QMH_Enqueue Message (poly).vi"("Priority Message? (F)"=TRUE, "error in"=w437, "Message"="Exit", "Message Queue in"=w438) -> ("error out"=w440:errorcluster)  [unwired: 6 in, 1 out]
            n160 = Merge Errors(w440) -> (w436:errorcluster)
          }
          frame "Exit" {
            w460 = 91  # 91: not all Exit messages will have an argument
            w463 = TRUE  # Stop the VI
            # "Release the message queue reference"
            # "Exit - Exit the application."
            n161 = Unbundle By Name(w445) -> ("UDP Conn. ID"=w444:refnum<k16>)
            n162 = Variant To Data(error in=w466, type=T7 {"Origin"="", "Module ID"=-1, "Exit via Stop Module Req?"=FALSE, "Wait for Module to stop?"=FALSE} ("Stop Argument"), Variant=w458) -> (data=w452:T7, error out=w459:errorcluster)
            n163 = property class="Mod Admin"(reference=w448) -> ("Accessors:Module ID"=w447:i32)  [unwired: 1 in, 2 out]
            n164 = call <vilib>:"Clear Errors.vi"("error in (no error)"=w459, "specific error code to clear (0: all)"=w460) -> ("error out"=w465:errorcluster)  [unwired: 4 in, 1 out]
            n165 = Not A Number/Path/Refnum?(number/path/refnum=w444) -> (NaN/Path/Refnum?=w446:bool)
            n166 = control-ref of="This VI"() -> (w455:refnum<vi>)
            n167 = case shown="False" w446 {
              tunnel: w444 -> [w468 _]
              tunnel: [w467 _] -> _
              frame False {
                n168 = UDP Close(connection ID=w468) -> (error out=w467:errorcluster)  [unwired: 1 in, 1 out]
              }
              frame True {
              }
            }
            n169 = call "Handle Exit.vi"("Stop Argument"=w452, "Module Admin in"=w448, "VI reference"=w455) -> ("error out"=w461:errorcluster, "Wait for Stop?"=w456:bool)  [unwired: 7 in]
            n170 = call-dynamic "Delacor_lib_QMH_Release Message Queue.vi"("error in"=w465, "Message Queue"=w464) -> ("error out"=w462:errorcluster)  [unwired: 9 in]
            n171 = property class="Mod Admin"(reference=w448) -> ("Accessors:Module ID"=w442:i32)  [unwired: 1 in, 2 out]
            n172 = Merge Errors(w461, w462) -> (w443:errorcluster)
            n173 = local read "listener ID"() -> (w454:refnum<k5>)
            n174 = Unbundle By Name(w452) -> ("Origin"=w451:string)
            n175 = call "Module Name--constant.vi"("Module ID"=w447) -> ("Module Name"=w450:string)  [unwired: 10 in]
            n176 = call "Error Reported.vi"("Error"=w443, "Module ID"=w442) -> ()  [unwired: 9 in, 1 out]
            n177 = Not A Number/Path/Refnum?(number/path/refnum=w454) -> (NaN/Path/Refnum?=w453:bool)
            n178 = case shown="False" w453 {
              tunnel: [w470 _] -> _
              tunnel: w454 -> [w469 _]
              frame False {
                n179 = TCP Close Connection(connection ID=w469) -> (error out=w470:errorcluster)  [unwired: 2 in, 1 out]
              }
              frame True {
              }
            }
            n180 = Format Into String(format string="%s stopped (%s)" ("Message"), w450, w451) -> ()  [unwired: 2 in, 2 out]
          }
          frame Default {
            # "'Default' case only runs if there is a message that isn't defined in any of the other cases.  Output a programming error."
            n181 = property class="Mod Admin"(reference=w472) -> ("Accessors:Module ID"=w471:i32)  [unwired: 1 in, 2 out]
            n182 = call "Module Name--constant.vi"("Module ID"=w471) -> ("Module Name"=w473:string)  [unwired: 10 in]
            n183 = xnode "Error Ring"("parameter 0"=w474, "parameter 1"=w473) -> ("error out"=w475:errorcluster)
          }
        }
        n184 = call-dynamic "Delacor_lib_QMH_Error Handler - Message Handling Loop.vi"("error in"=w340, "Message Queue in"=w331) -> ("dup error in"=w330:errorcluster)  [unwired: 8 in, 1 out]
      }
    }
    frame Error {
      n185 = call "Synchronize Caller Events.vi"("Module Admin"=w490) -> ("Module Admin out"=w489:refnum<class "Delacor_lib_QMH_Cloneable Module Admin.lvclass">)  [unwired: 9 in, 1 out]
      n186 = property class="Mod Admin"(reference=w489) -> ("Accessors:Module ID"=w488:i32)  [unwired: 1 in, 2 out]
      n187 = call-dynamic "Delacor_lib_QMH_Release Message Queue.vi"("Message Queue"=w486) -> ()  [unwired: 10 in, 1 out]
      n188 = call-dynamic "Delacor_lib_QMH_Release Message Queue.vi"("Message Queue"=w485) -> ()  [unwired: 10 in, 1 out]
      n189 = call "Module Name--constant.vi"("Module ID"=w488) -> ("Module Name"=w493:string)  [unwired: 10 in]
      n190 = Format Into String(format string="An error occurred during initialization. %s is no longer running.", w493) -> (resulting string=w491:string)  [unwired: 2 in, 1 out]
      n191 = call "Error Reported.vi"("Additional Information"=w491, "Error"=w494, "Module ID"=w488) -> ()  [unwired: 8 in, 1 out]
    }
  }
  n192 = Merge Errors(w25, w24) -> (w26:errorcluster)
  n193 = call "Close Module.vi"("error in (no error)"=w26, "Wait for stop?"=w16, "Module Admin in"=w18) -> ("error out"=w10:errorcluster, "External Launch"=w14:bool, "Module Admin out"=w17:refnum<class "Delacor_lib_QMH_Cloneable Module Admin.lvclass">)  [unwired: 6 in]
  n194 = Unregister For Events(event registration refnum=w8, error in=w10) -> (error out=w9:errorcluster)
  n195 = Unregister For Events(event registration refnum=w22, error in=w9) -> (error out=w15:errorcluster)
  "error out" <- w15
  n196 = local write "Module Admin"(w17) -> ()
  n197 = case "External Launch?" shown="True" w14 {
    tunnel: w15 -> [_ w496]
    frame False {
    }
    frame True {
      n198 = case shown="No Error" w496 {
        frame No Error {
          n199 = invoke class="VI" method="FP.Close"() -> ()  [unwired: 3 in, 3 out]
        }
        frame Error {
          n200 = invoke class="VI" method="FP.Open"("Activate"=TRUE ("Activate?")) -> ()  [unwired: 4 in, 5 out]
        }
      }
    }
  }
